vi "Port to Read.vi"(8 "error in (no error)":errorcluster, 10 "Port to Read":dbl, 11 "NXP in":refnum<class "NXP.lvclass">) -> (0 "error out":errorcluster, 3 "NXP out":refnum<class "NXP.lvclass">)   [LabVIEW 2020, in "NXP.lvclass"]
doc: "Port to read es el vi donde se manda al microcontrolador los datos del puerto que se desea leer"
uses:
  NXP.lvclass
  NXP.lvclass/NXP.ctl
  45f88905-1da1-4c33-880c-58c6d610e7d8.vi
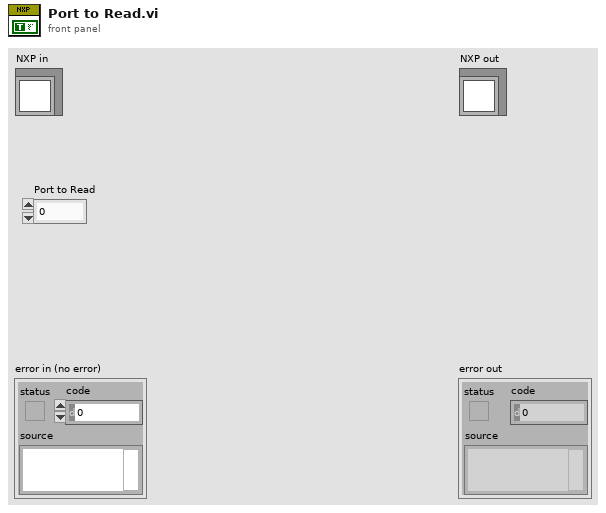
[diagram p1: front panel]
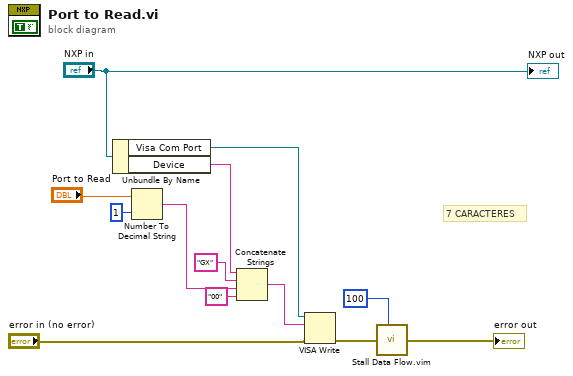
[diagram p0: block diagram]
diagram:
  # "7 CARACTERES"
  n1 = Unbundle By Name("NXP in") -> ("Visa Com Port"=w12:refnum<visa-resource-name>, "Device"=w10:string)
  n2 = Number To Decimal String(number="Port to Read", width (-)=i16 1) -> (decimal integer string=w9:string)
  n3 = Concatenate Strings(w10, "GX" ("string"), w9, "00" ("string")) -> (w11:string)
  n4 = VISA Write(VISA resource name=w12, write buffer=w11, error in (no error)="error in (no error)") -> (error out=w13:errorcluster)  [unwired: 2 out]
  n5 = call "Stall Data Flow.vim"("value in"=w13, "milliseconds to wait"=u32 100) -> ("value out"=→"error out":errorcluster)  [unwired: 1 out]
  "NXP out" <- "NXP in"
